vi "Test Parse with missing attribute in JSON.vi"(11 "Test Case In":refnum<class "Test Strict Find Items as LV Type.lvclass">) -> (0 "error out":errorcluster, 3 "Test Case Out":refnum<class "Test Strict Find Items as LV Type.lvclass">)   [LabVIEW 2024, in "Test Strict Find Items as LV Type.lvclass"]
uses:
  Test Strict Find Items as LV Type.lvclass
  Test Strict Find Items as LV Type.lvclass/Test Strict Find Items as LV Type.ctl
  7860c969-8ea9-4e34-a02d-68fc78db45ce.vi
  <vilib>/Astemes/LUnit/Test Case.lvclass
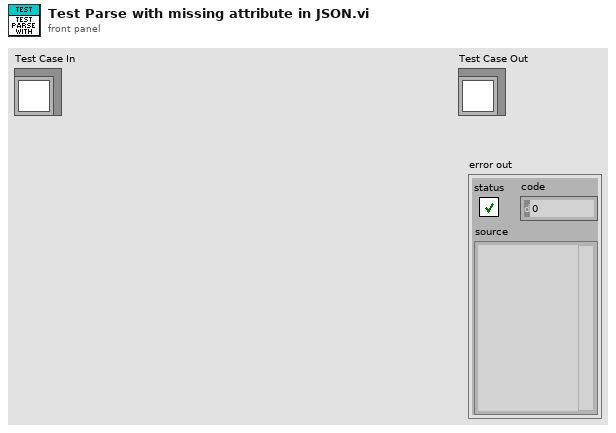
[diagram p1: front panel]
types:
  T1 = cluster{"Instr Ident":string, "Enabled":bool, "Value":dbl}
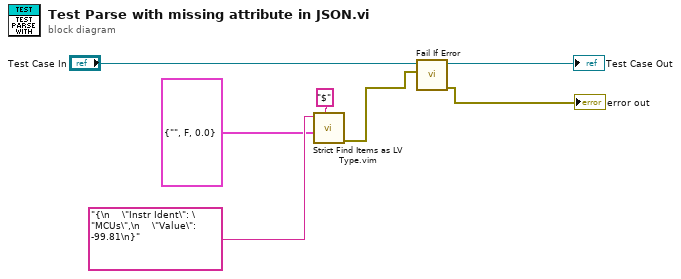
[diagram p0: block diagram]
diagram:
  n1 = call "Strict Find Items as LV Type.vim"("$Path or Item Name"="$", "Data Type and Default Value"=T1 {"Instr Ident"="", "Enabled"=FALSE, "Value"=0.0}, "<JSON>"="{\n    \"Instr Ident\": \"MCUs\",\n    \"Value\": -99.81\n}") -> ("error out"=w1:errorcluster)  [unwired: 6 in, 2 out]
  n2 = call <vilib>:"Fail If Error.vi"("Assert error"=w1, "LUnit Test Case In"="Test Case In") -> ("error out"=→"error out":errorcluster, "LUnit Test Case Out"=→"Test Case Out":refnum<class "Test Strict Find Items as LV Type.lvclass">)  [unwired: 8 in]
